vi "DtOLReadSingleU32.vi"(8 "error in (no error)":errorcluster, 9 "Timeout":dbl=10.0, 11 "Task in":i32) -> (0 "error out":errorcluster, 2 "Data Out":u32, 3 "Task out":i32)   [LabVIEW 2016]
doc: "Reads a single sample from a single virtual channel of a task you specify, and returns the data as an unsigned 32-bit number.\n\nThis VI is typically used with tasks that were created using the Analog Input - Raw instance of the DtOLCreateTask VI."
uses:
  <userlib>/LV-Link3/DtLvLink.lvlib
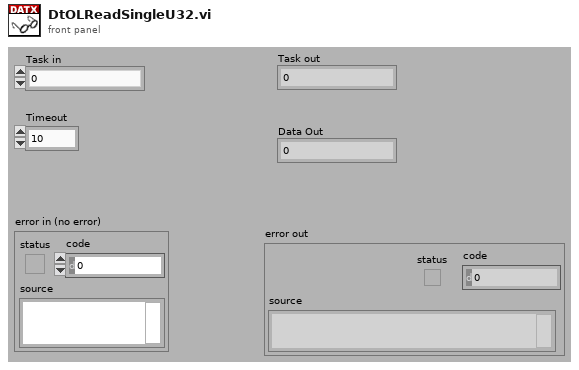
[diagram p1: front panel]
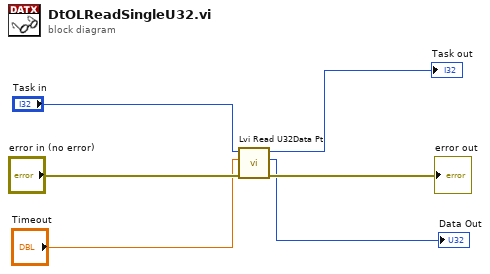
[diagram p0: block diagram]
diagram:
  n1 = call <userlib>:"Lvi Read U32Data Pt.vi"("error in (no error)"="error in (no error)", "timeout"="Timeout", "TaskRef"="Task in") -> ("error out"=→"error out":errorcluster, "DataBuf"=→"Data Out":u32, "TaskRef out"=→"Task out":i32)  [unwired: 5 in, 1 out]
